vi "CalcSampleRVErrorSplitterBox.vi"(0 "Source Voltage (V)":dbl format="%#_13g", 5 "Sample Current (A)":dbl format="%#_13g", 7 "Sample Current StDev (A)":dbl format="%#_13g", 9 "Rl":dbl format="%#_13g", 11 "Rp":dbl format="%#_13g") -> (4 "Sample Voltage StDev (V)":dbl, 15 "Sample Resistance StDev (Ohms)":dbl)   [LabVIEW 2016]
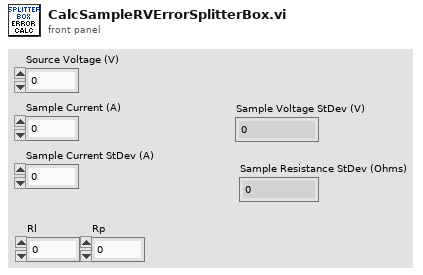
[diagram p1: front panel]
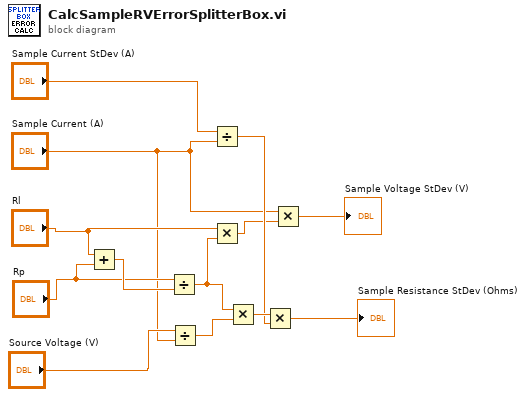
[diagram p0: block diagram]
diagram:
  n1 = Add(x="Rl", y="Rp") -> (x+y=w13:dbl)
  n2 = Divide(x="Rp", y=w13) -> (x/y=w5:dbl)
  n3 = Divide(x="Source Voltage (V)", y="Sample Current (A)") -> (x/y=w10:dbl)
  n4 = Divide(x="Sample Current StDev (A)", y="Sample Current (A)") -> (x/y=w7:dbl)
  n5 = Multiply(x="Rl", y=w5) -> (x*y=w3:dbl)
  n6 = Multiply(x=w5, y=w10) -> (x*y=w8:dbl)
  n7 = Multiply(x=w8, y=w7) -> (x*y=→"Sample Resistance StDev (Ohms)":dbl)
  n8 = Multiply(x="Sample Current (A)", y=w3) -> (x*y=→"Sample Voltage StDev (V)":dbl)
